vi "Write_EQ_and_Enable.vi"(4 "error in":errorcluster, 7 "gRPC ID in":T3) -> (0 "error out":errorcluster, 1 "Bypass Response":T1, 2 "EQ Response":T2, 3 "gRPC ID out":T3)   [LabVIEW 2024]
uses:
  <vilib>/gRPC/LabVIEW gRPC Library/Shared/grpcId.ctl
  RPC Messages/rfcontrol_SetRFDCCalibrationCoefficientsResponse.ctl
  RPC Messages/rfcontrol_SetRFDCCalibrationCoefficientsRequest.ctl
  RPC Messages/rfcontrol_RFDC.ctl
  <vilib>/Utility/file.llb/Read Delimited Spreadsheet (DBL).vi
  FlexSDR_gRPC_client.lvlib
  RPC Messages/rfcontrol_SetRFDCCalibrationBypassRequest.ctl
  <vilib>/gRPC/LabVIEW gRPC Library/grpc-lvsupport-release.lvlib
  RPC Messages/rfcontrol_SetRFDCCalibrationBypassResponse.ctl
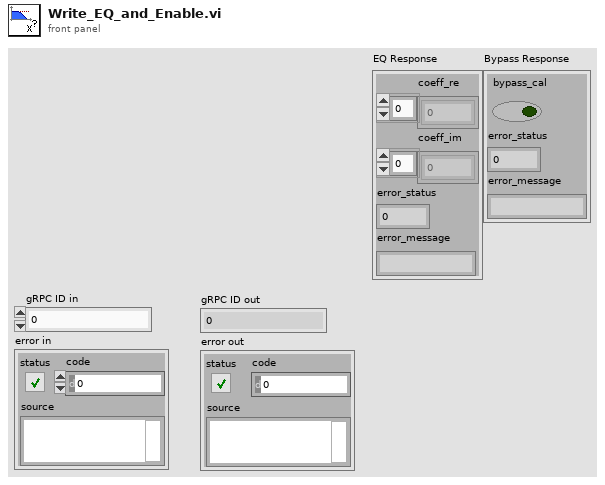
[diagram p1: front panel]
types:
  T1 = typedef "FlexSDR_gRPC_client.lvlib/rfcontrol_SetRFDCCalibrationBypassResponse.ctl" = cluster{"bypass_cal":bool, "error_status":i32, "error_message":string}
  T2 = typedef "FlexSDR_gRPC_client.lvlib/rfcontrol_SetRFDCCalibrationCoefficientsResponse.ctl" = cluster{"coeff_re":i32[], "coeff_im":i32[], "error_status":i32, "error_message":string}
  T3 = typedef "grpc-lvsupport-release.lvlib/grpcId.ctl" = u64
  T4 = typedef "FlexSDR_gRPC_client.lvlib/rfcontrol_SetRFDCCalibrationBypassRequest.ctl" = cluster{"device_id":string, "rfdc":T5, "bypass_cal":bool, "error_queue_populate":bool}
  T5 = typedef "FlexSDR_gRPC_client.lvlib/rfcontrol_RFDC.ctl" = enum32{"TX1", "TX2", "TX3", "TX4", "TX5", "TX6", "TX7", "TX8", "RX1", "RX2", "RX3", "RX4", "RX5", "RX6", "RX7", "RX8", "WRX1", "WRX2"}
  T6 = typedef "FlexSDR_gRPC_client.lvlib/rfcontrol_SetRFDCCalibrationCoefficientsRequest.ctl" = cluster{"device_id":string, "rfdc":T5, "coeff_re":i32[], "coeff_im":i32[], "error_queue_populate":bool}
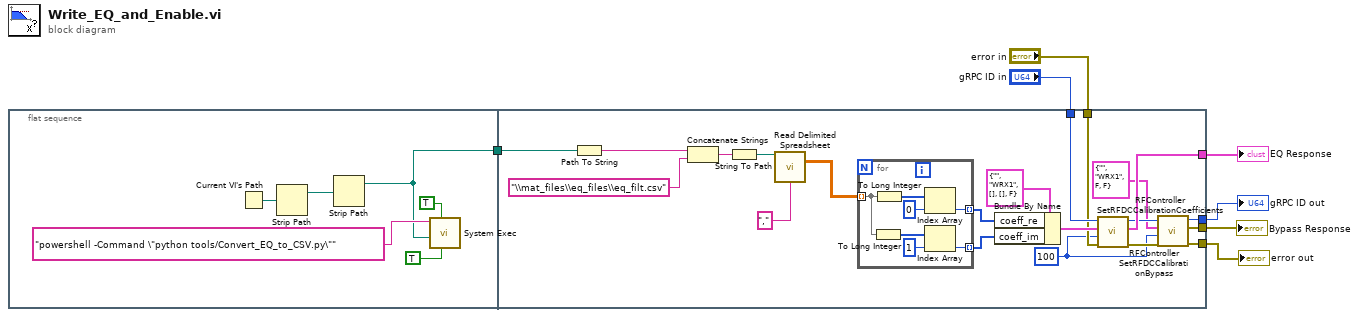
[diagram p0: block diagram]
diagram:
  n1 = flat-sequence {
    tunnel: [w8] -> w7
    tunnel: w7 -> [w34]
    tunnel: "gRPC ID in" -> [w23]
    tunnel: "error in" -> [w22]
    tunnel: [w21] -> w4
    tunnel: [w16] -> w1
    tunnel: [w15] -> w2
    tunnel: [w14] -> w3
    frame #0 {
      n2 = Current VI's Path() -> (path=w12:path)
      n3 = Strip Path(path=w12) -> (stripped path=w11:path)  [unwired: 1 out]
      n4 = Strip Path(path=w11) -> (stripped path=w8:path)  [unwired: 1 out]
      n5 = call <vilib>:"System Exec.vi"("run minimized? (F)"=TRUE, "wait until completion? (T)"=TRUE, "working directory"=w8, "command line"="powershell -Command \"python tools/Convert_EQ_to_CSV.py\"") -> ()  [unwired: 4 in, 4 out]
    }
    frame #1 {
      w18 = 100 ("timeout (ms)")
      n6 = Path To String(path=w34) -> (string=w33:string)
      n7 = Concatenate Strings(w33, "\\mat_files\\eq_files\\eq_filt.csv" ("string")) -> (w31:string)
      n8 = String To Path(string=w31) -> (path=w30:path)
      n9 = call-poly <vilib>:"Read Delimited Spreadsheet.vi"("file path (dialog if empty)"=w30, "delimiter (\\t)"="," ("delimiter (\\t)")) -> ("all rows"=w28:dbl[][])  [unwired: 8 in, 5 out]
      n10 = for {
        tunnel: w28 -> [w36] mode=indexing
        tunnel: [w39] -> w26 mode=indexing
        tunnel: [w38] -> w25 mode=indexing
        n11 = To Long Integer(number=w36) -> (32bit integer=w35:i32[])
        n12 = To Long Integer(number=w36) -> (32bit integer=w37:i32[])
        n13 = Index Array(array=w37, index=0) -> (element=w39:i32)
        n14 = Index Array(array=w35, index=1) -> (element=w38:i32)
      }
      n15 = Bundle By Name(cluster=T6 {"device_id"="", "rfdc"=enum."WRX1", "coeff_re"=[], "coeff_im"=[], "error_queue_populate"=FALSE} ("Request Data"), "coeff_re"=w26, "coeff_im"=w25) -> (w24:T6)
      n16 = call "RFController SetRFDCCalibrationCoefficients.vi"("error in"=w22, "timeout (ms)"=w18, "Request Data"=w24, "gRPC ID"=w23) -> ("error out"=w20:errorcluster, "Response Data"=w21:T2, "gRPC ID out"=w19:T3)  [unwired: 5 in]
      n17 = call "RFController SetRFDCCalibrationBypass.vi"("error in"=w20, "timeout (ms)"=w18, "Request Data"=T4 {"device_id"="", "rfdc"=enum."WRX1", "bypass_cal"=FALSE, "error_queue_populate"=FALSE}, "gRPC ID"=w19) -> ("error out"=w16:errorcluster, "Response Data"=w14:T1, "gRPC ID out"=w15:T3)  [unwired: 5 in]
    }
  }
  "gRPC ID out" <- w2
  "error out" <- w1
  "EQ Response" <- w4
  "Bypass Response" <- w3
